vi "SLL DE Get the order of Virtual Channels Ver1.vi"(8 "error in (no error)":errorcluster, 9 "Channel Array":cluster{"Device Channel List":string[]}[](array[cluster]), 11 "Virtial Channels Info":string[](array[string])) -> (0 "error out":errorcluster, 3 "Channel Order":i32[](array[numeric]))   [LabVIEW 2013]
doc: "Copyright © 2005, Soliton Technologies.\nAll rights reserved."
uses:
  Instance           1 41Saved   Get the order of Virtual Channels .vi
panel:
  out "Virtial Channels Info out":string[](array[string])
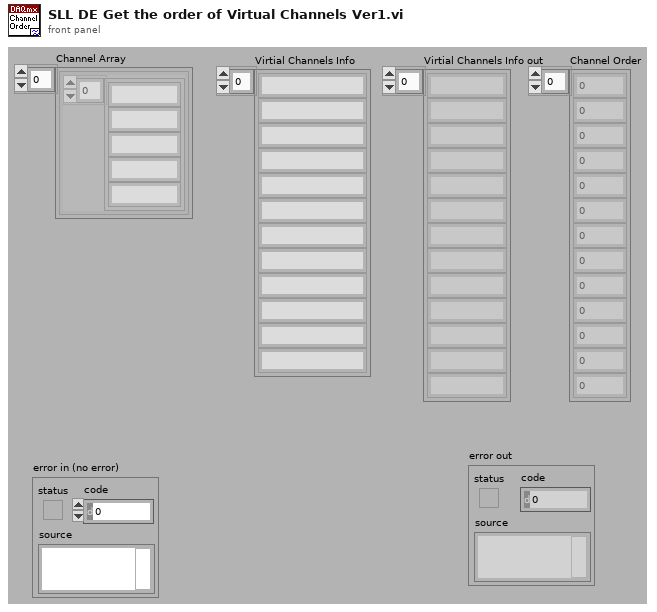
[diagram p1: front panel]
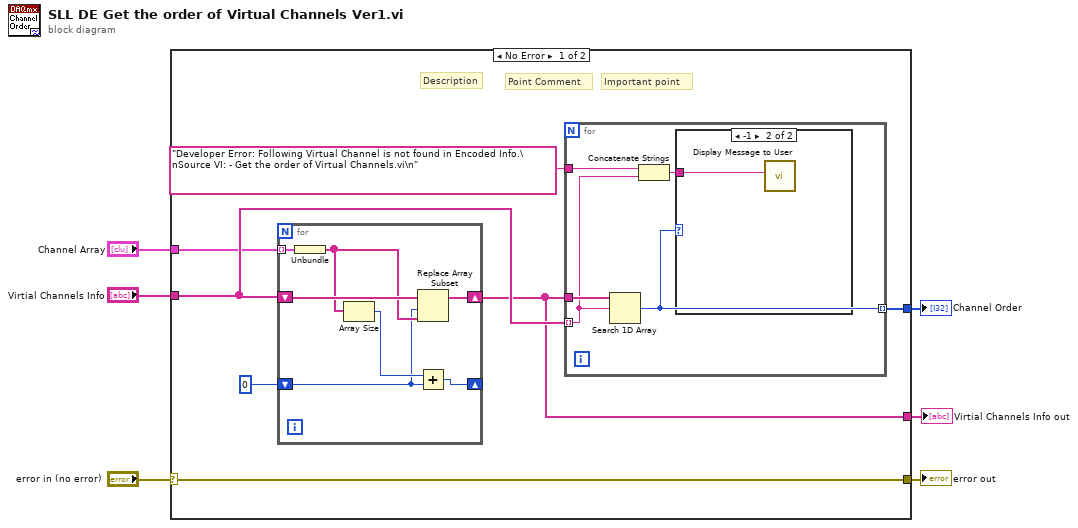
[diagram p0: block diagram]
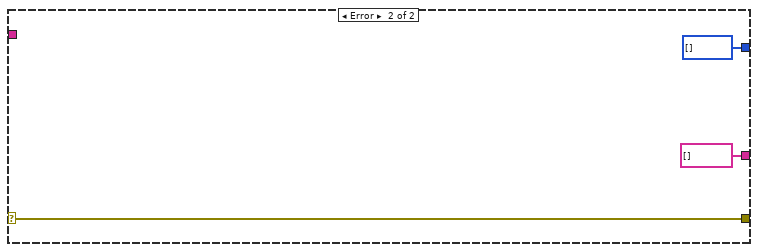
[diagram p3: hidden frame]
diagram:
  n1 = case shown="No Error" "error in (no error)" {
    selector: "error in (no error)" -> [w13 w29]
    tunnel: [w13 w29] -> w5
    tunnel: "Virtial Channels Info" -> [w11 _]
    tunnel: [w9 i32[] []] -> w3
    tunnel: "Channel Array" -> [w8 _]
    tunnel: [w7 string[] [] ("Virtial Channels Info")] -> w1
    frame No Error {
      # "Point Comment"
      # "Important point"
      # "Description"
      n2 = for {
        shift-right: [w24] -> w7
        shift-left: w11 -> [w26]
        shift-right: [w25] -> _
        shift-left: 0 ("Virtual Channel Name") -> [w20]
        tunnel: w8 -> [w23] mode=indexing
        n3 = Unbundle(w23) -> ("Device Channel List"=w22:string[])
        n4 = Array Size(array=w22) -> (size(s)=w21:i32)
        n5 = Replace Array Subset(array=w26, new element=w22, index=w20) -> (w24:string[])
        n6 = Add(x=w21, y=w20) -> (x+y=w25:i32)
      }
      n7 = for {
        tunnel: w7 -> [w18]
        tunnel: w11 -> [w15] mode=indexing
        tunnel: [w17] -> w9 mode=indexing
        tunnel: "Developer Error: Following Virtual Channel is not found in Encoded Info.\nSource VI: - Get the order of Virtual Channels.vi\n" ("Virtual Channel Name") -> [w16]
        n8 = Search 1D Array(1D array=w18, element=w15) -> (index of element=w17:i32)  [unwired: 1 in]
        n9 = Concatenate Strings(w16, w15) -> (w14:string)
        n10 = case shown="-1" w17 {
          tunnel: w14 -> [_ w19]
          frame 0, Default {
          }
          frame -1 {
            n11 = call "Display Message to User"("Message"=w19) -> ()  [unwired: 9 in, 2 out]
          }
        }
      }
    }
    frame Error {
    }
  }
  "error out" <- w5
  "Channel Order" <- w3
  "Virtial Channels Info out" <- w1
